vi "merge_Count Down.vi"   [LabVIEW 2017, in "NI_FunctionBlockMergeVIs.lvlib"]
doc: "Counts down from the number you specify using the <B>preset value</B> input. The <B>counter value</B> output decrements on each rising edge of the <B>count down</B> input. When <B>counter value</B> reaches zero, <B>done</B> returns TRUE."
uses:
  <vilib>/functionblocks/NI_FunctionBlockMergeVIs.lvlib
  <vilib>/functionblocks/FB Core/FB Core.xnode
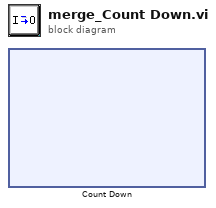
[diagram p0: block diagram]
diagram:
  n1 = xnode "Count Down"() -> ()  [unwired: 4 in, 3 out]
